vi "Step_2_Ans_PS.vi"   [LabVIEW 2012]
types:
  T1 = typedef "BotSpeak_Control.ctl" = cluster{"Address":string, "Reply EOF":string, "Hardware":string, "Retries":i8, "Timeout":i32}
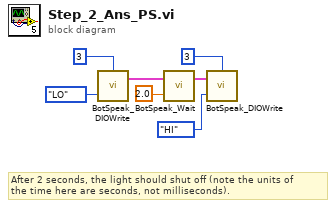
[diagram p0: block diagram]
diagram:
  # "After 2 seconds, the light should shut off (note the units of\nthe time here are seconds, not milliseconds)."
  n1 = call <userlib>:"BotSpeak_DIOWrite.vi"("State"=enum32{"LO", "HI"}."LO", "DIO Line"=u32 3) -> ("Bot Settings"=w1:T1)  [unwired: 1 in, 1 out]
  n2 = call <userlib>:"BotSpeak_Wait.vi"("Wait (sec)"=2.0, "Bot Settings"=w1) -> ("Bot Settings"=w2:T1)  [unwired: 1 in]
  n3 = call <userlib>:"BotSpeak_DIOWrite.vi"("State"=enum32{"LO", "HI"}."HI", "Bot Settings"=w2, "DIO Line"=u32 3) -> ()  [unwired: 2 out]
